vi "_StrTable to LogicCfg.vi"(8 "error in (no error)":errorcluster, 11 "CfgTable in":string[][](array[string])) -> (0 "error out":errorcluster, 3 "Array 2":T1[](array[typedef]))   [LabVIEW 2017, in "TagDB RefManager.lvlib"]
uses:
  TagDB RefManager.lvlib
  Typedef/RefMgr-Logic-State.ctl
  Typedef/RefMgr-StateChangeType.ctl
  627ab74d-fd43-4f3b-ae31-bc93842384ce.vi
  618c08d7-4f0e-4c08-8238-d9ecc43b0f03.vi
  480c0bf6-53d7-4c76-b845-d201bd49c9a1.vi
  8c544a5d-1875-4e5e-ad53-38d52155ea8b.vi
  <userlib>/_OpenG.lib/string/string.llb/Trim Whitespace (String Array)__ogtk.vi
  <userlib>/NEVSTOP-Programming-Palette/Configuration/ClusterCfgTable/Parse CfgTable(with DataName).vi
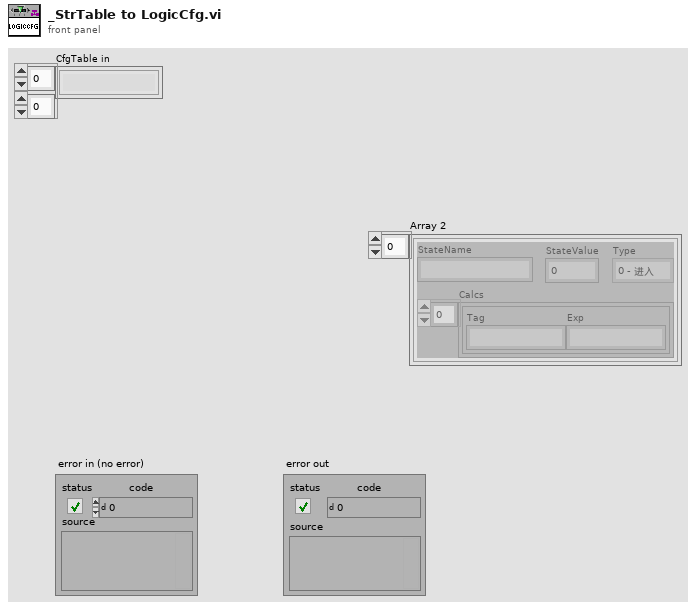
[diagram p1: front panel]
types:
  T1 = typedef "TagDB RefManager.lvlib/RefMgr-Logic-State.ctl" = cluster{"StateName":string, "StateValue":i32, "Type":T2, "Calcs":cluster{"Tag":string, "Exp":string}[]}
  T2 = typedef "TagDB RefManager.lvlib/RefMgr-StateChangeType.ctl" = enum16{"0 - 进入", "1 - 等于", "2 - 退出"}
  T3 = cluster{"StateName":string, "StateName 2":string, "StateValue":i32, "Type":T2}
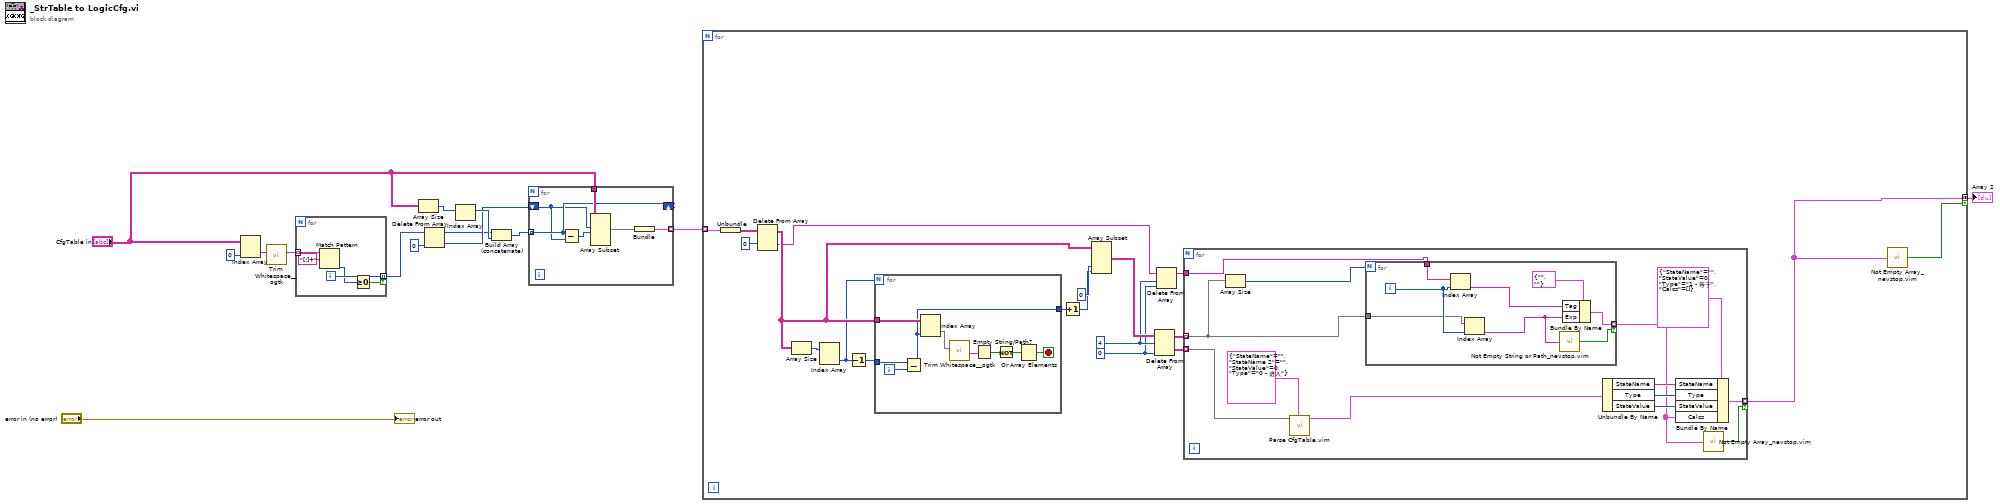
[diagram p0: block diagram]
diagram:
  n1 = Index Array(array="CfgTable in", index (col)=0 ("disabled index (col)")) -> (element=w4:string[])  [unwired: 1 in]
  n2 = call-poly <userlib>:"Trim Whitespace__ogtk.vi"("String in"=w4) -> ("String out"=w6:string[])  [unwired: 6 in]
  n3 = for {
    tunnel: w6 -> [w19] mode=indexing
    tunnel: [w17] -> w7 mode=indexing if=w15
    i -> [w17]
    n4 = Match Pattern(string=w19, regular expression="[!]+") -> (offset past match=w16:i32)  [unwired: 1 in, 3 out]
    n5 = Greater Or Equal To 0?(x=w16) -> (x >= 0?=w15:bool)
  }
  n6 = Array Size(array="CfgTable in") -> (size(s)=w12:i32[])
  n7 = Delete From Array(array=w7, index=0) -> (deleted portion=w10:i32, array with subset deleted=w9:i32[])  [unwired: 1 in]
  n8 = Index Array(array=w12) -> (element=w13:i32)  [unwired: 1 in]
  n9 = Build Array (concatenate)(w9, w13) -> (w11:i32[])
  n10 = for {
    tunnel: "CfgTable in" -> [w25]
    tunnel: w11 -> [w22] mode=indexing
    tunnel: [w23] -> w8 mode=indexing
    shift-right: [w22] -> _
    shift-left: w10 -> [w20]
    n11 = Subtract(x=w22, y=w20) -> (x-y=w21:i32)
    n12 = Array Subset(array=w25, index (row)=w20, length (row)=w21) -> (w24:string[][])  [unwired: 2 in]
    n13 = Bundle(w24) -> (w23:cluster{string[][]})  [unwired: 1 in]
  }
  n14 = for {
    tunnel: w8 -> [w44] mode=indexing
    tunnel: [w26] -> w1 mode=concatenating if=w27
    w28 = 0 ("disabled index (col)")
    w29 = 4 ("length")
    n15 = Unbundle(w44) -> (w43:string[][])
    n16 = Delete From Array(array=w43, index (row)=0 ("disabled index (col)")) -> (deleted portion=w31:string[], array with subset deleted=w39:string[][])  [unwired: 2 in]
    n17 = Array Size(array=w39) -> (size(s)=w41:i32[])
    n18 = Index Array(array=w41) -> (element #2=w36:i32)  [unwired: 2 in, 1 out]
    n19 = Decrement(x=w36) -> (x-1=w40:i32)
    n20 = for {
      N: w36 -> [_]
      tunnel: w39 -> [w74]
      tunnel: w40 -> [w73]
      tunnel: [w67] -> w38
      i -> [w68]
      stop <- w69 stop-if-true
      n21 = Subtract(x=w73, y=w68) -> (x-y=w67:i32)
      n22 = Index Array(array=w74, index (col)=w67) -> (element=w72:string[])  [unwired: 1 in]
      n23 = call-poly <userlib>:"Trim Whitespace__ogtk.vi"("String in"=w72) -> ("String out"=w71:string[])  [unwired: 6 in]
      n24 = Empty String/Path?(string/path=w71) -> (empty?=w70:bool[])
      n25 = Not(x=w70) -> (.not. x?=w66:bool[])
      n26 = Or Array Elements(Boolean array=w66) -> (logical OR=w69:bool)
    }
    n27 = Increment(x=w38) -> (x+1=w35:i32)
    n28 = Array Subset(array=w39, index (col)=0 ("index"), length (col)=w35) -> (w34:string[][])  [unwired: 2 in]
    n29 = Delete From Array(array=w34, length=w29, index (col)=w28) -> (deleted portion=w33:string[][], array with subset deleted=w32:string[][])  [unwired: 1 in]
    n30 = Delete From Array(array=w31, length=w29, index=w28) -> (array with subset deleted=w30:string[])  [unwired: 1 out]
    n31 = for {
      tunnel: w33 -> [w57] mode=indexing
      tunnel: w32 -> [w51] mode=indexing
      tunnel: w30 -> [w50]
      tunnel: [w49] -> w26 mode=indexing if=w47
      n32 = Array Size(array=w51) -> (size(s)=w46:i32)
      n33 = call "Parse CfgTable.vim"("Cluster Configuration Typedef"=T3 {"StateName"="", "StateName 2"="", "StateValue"=0, "Type"=enum."0 - 进入"} ("Cluster"), "CfgTable Row"=w57) -> ("Cluster Configuration Out"=w55:T3)  [unwired: 8 in, 1 out]
      n34 = for {
        N: w46 -> [_]
        tunnel: w51 -> [w59]
        tunnel: w50 -> [w65]
        tunnel: [w62] -> w48 mode=indexing if=w61
        i -> [w60]
        n35 = Index Array(array=w65, index=w60) -> (element=w63:string)
        n36 = Index Array(array=w59, index=w60) -> (element=w58:string)
        n37 = call "Not Empty String or Path_nevstop.vim"("String"=w58) -> ("not empty?"=w61:bool)
        n38 = Bundle By Name(cluster=cluster{"Tag":string, "Exp":string} {"Tag"="", "Exp"=""} ("Cluster"), "Tag"=w63, "Exp"=w58) -> (w62:cluster{"Tag":string, "Exp":string})
      }
      n39 = Unbundle By Name(w55) -> ("StateName"=w52:string, "Type"=w53:T2, "StateValue"=w54:i32)
      n40 = Bundle By Name(cluster=T1 {"StateName"="", "StateValue"=0, "Type"=enum."1 - 等于", "Calcs"=[]} ("Cluster"), "StateName"=w52, "Type"=w53, "StateValue"=w54, "Calcs"=w48) -> (w49:T1)
      n41 = call "Not Empty Array_nevstop.vim"("Array"=w48) -> ("not empty?"=w47:bool)
    }
    n42 = call "Not Empty Array_nevstop.vim"("Array"=w26) -> ("not empty?"=w27:bool)
  }
  "Array 2" <- w1
  "error out" <- "error in (no error)"
